vi "Delete CDS.vi"(8 "error in (no error)":errorcluster, 11 "Assert VI Path":path) -> (0 "error out":errorcluster, 2 "Found?":bool)   [LabVIEW 2018]
doc: "Deletes a specified conditional disable structure from the target block diagram"
uses:
  <vilib>/Utility/traverseref.llb/TRef TravTarget.ctl
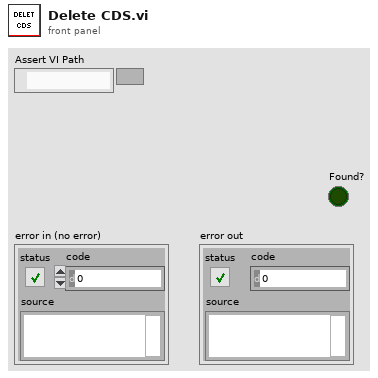
[diagram p1: front panel]
types:
  T1 = typedef "TRef TravTarget.ctl" = enum16{"FP", "BD", "Other"}
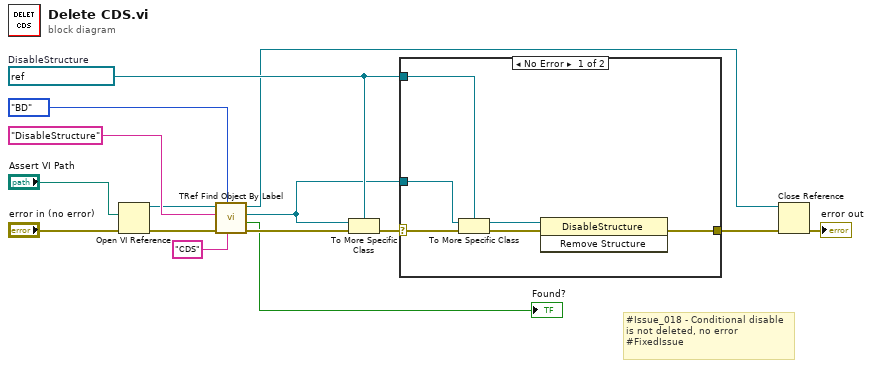
[diagram p0: block diagram]
diagram:
  w3 = refnum<vi> refnum  # DisableStructure
  # "#Issue_018 - Conditional disable is not deleted, no error\n#FixedIssue"
  n1 = Open VI Reference(vi path="Assert VI Path", error in (no error)="error in (no error)") -> (vi reference=w8:refnum<vi>, error out=w11:errorcluster)  [unwired: 4 in]
  n2 = call <vilib>:"TRef Find Object By Label.vi"("Label"="CDS", "Traverse Target"=TRef_TravTarget."BD", "error in (no error)"=w11, "Class Name"="DisableStructure", "VI Ref"=w8) -> ("error out"=w6:errorcluster, "Found?"=→"Found?":bool, "Found Obj Ref"=w2:refnum<vi>, "dup VI Ref"=w1:refnum<vi>)  [unwired: 3 in]
  n3 = To More Specific Class(target class=w3, reference=w2, error in=w6) -> (error out=w5:errorcluster)  [unwired: 1 out]
  n4 = case shown="No Error" w5 {
    selector: w5 -> [w20 w22]
    tunnel: [w21 w22] -> w12
    tunnel: w3 -> [w18 _]
    tunnel: w2 -> [w17 _]
    frame No Error {
      n5 = To More Specific Class(target class=w18, reference=w17, error in=w20) -> (specific class reference=w16:refnum<vi>, error out=w19:errorcluster)
      n6 = invoke class="DisableStructure" method="Remove Structure"(reference=w16, error in=w19) -> (error out=w21:errorcluster)  [unwired: 1 in, 2 out]
    }
    frame Error {
      # "This should never happen as it should only be used on a vi with the correct conditional disable structure"
    }
  }
  n7 = Close Reference(reference=w1, error in (no error)=w12) -> (error out=→"error out":errorcluster)
